vi "get Renderer.vi"(11 "Renderer in":refnum<class "Renderer.lvclass">) -> (3 "Renderer":u32 format="%.0x")   [LabVIEW 2021, in "Renderer.lvclass"]
uses:
  Renderer.lvclass
  Renderer.lvclass/Renderer.ctl
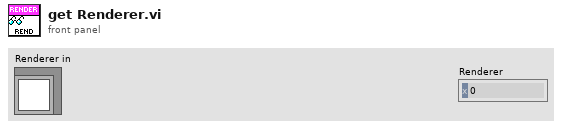
[diagram p1: front panel]
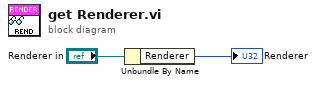
[diagram p0: block diagram]
diagram:
  n1 = Unbundle By Name("Renderer in") -> ("Renderer"=→"Renderer":u32)
